vi "ListUser.vi"(1 "UserLibFile":path) -> (0 "Users":string[][](array[string]))   [LabVIEW 2020]
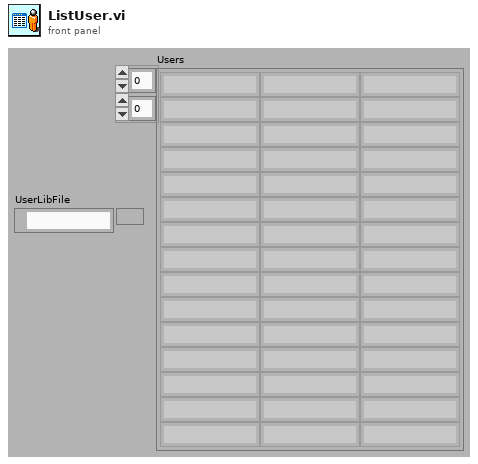
[diagram p1: front panel]
types:
  T1 = enum16{"open", "replace", "create", "open or create", "replace or create", "replace or create with confirmation"}
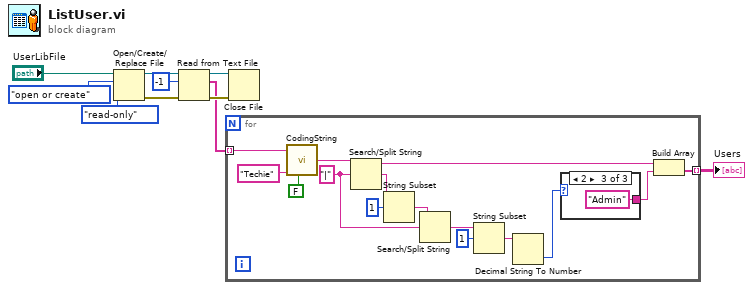
[diagram p0: block diagram]
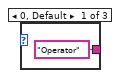
[diagram p2: hidden frame]
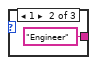
[diagram p3: hidden frame]
diagram:
  n1 = Open/Create/Replace File(file path (use dialog)="UserLibFile", operation (0:open)=T1."open or create", access (0:read/write)=enum16{"read/write", "read-only", "write-only"}."read-only") -> (refnum out=w6:refnum<file>, error out=w5:errorcluster)  [unwired: 1 in, 3 out]
  n2 = Read from Text File(file (use dialog)=w6, count=-1, error in=w5) -> (refnum out=w8:refnum<file>, text=w3:string[], error out=w7:errorcluster)  [unwired: 2 out]
  n3 = for {
    tunnel: w3 -> [w24] mode=indexing
    tunnel: [w25] -> w2 mode=indexing
    w20 = "|" ("search string/char (-)")
    n4 = call "CodingString.vi"("InputStr"=w24, "key"="Techie", "Coding(T)?"=FALSE) -> ("Output"=w14:string)  [unwired: 2 out]
    n5 = Search/Split String(string=w14, search string/char (-)=w20) -> (substring before match=w13:string, match + rest of string=w17:string)  [unwired: 2 out]
    n6 = String Subset(string=w17, offset (0)=1) -> (substring=w16:string)  [unwired: 1 out]
    n7 = Search/Split String(string=w16, search string/char (-)=w20) -> (match + rest of string=w19:string)  [unwired: 3 out]
    n8 = String Subset(string=w19, offset (0)=1) -> (substring=w21:string)  [unwired: 1 out]
    n9 = Decimal String To Number(string=w21) -> (number=w12:i32)  [unwired: 3 out]
    n10 = case shown="2" w12 {
      tunnel: ["Operator" ("key") "Engineer" ("key") "Admin" ("key")] -> w11
      frame 0, Default {
      }
      frame 1 {
      }
      frame 2 {
      }
    }
    n11 = Build Array(w13, w11) -> (w25:string[])
  }
  "Users" <- w2
  n12 = Close File(refnum=w8, error in=w7) -> ()  [unwired: 2 out]
